vi "Test_Connection.vi"() -> ()   [LabVIEW 2024]
uses:
  <vilib>/LabVIEW Open Source Project/MQTT Control Packets/Control Packets/CONNECT/ConnectFlags -- cluster.ctl
  <vilib>/LabVIEW Open Source Project/MQTT Control Packets/Control Packets/CONNACK/Connect Return Code -- enum.ctl
  <vilib>/LabVIEW Open Source Project/MQTT Secured TCP Connection/Connection.SecuredTCP/Connection.TCP-TLS.lvclass/Connection.TCP-TLS.ctl
  dcce8393-494f-4dd8-9f2c-9d268c5ade08.vi
  <vilib>/LabVIEW Open Source Project/MQTT Secured TCP Connection/Connection.SecuredTCP/Read trusted entities.vi
  <vilib>/LabVIEW Open Source Project/MQTT Secured TCP Connection/Connection.SecuredTCP/Write trusted entities.vi
  <vilib>/LabVIEW Open Source Project/MQTT Secured TCP Connection/Connection.SecuredTCP/Connection.TCP-TLS.lvclass
  C:/Program Files (x86)/National Instruments/LabVIEW 2024/vi.lib/LabVIEW Open Source Project/Connection/Connection/Connection.lvclass
  <vilib>/LabVIEW Open Source Project/MQTT Client/Client class/Client.lvclass
  C:/Program Files (x86)/National Instruments/LabVIEW 2024/vi.lib/LabVIEW Open Source Project/MQTT Connection/MQTT_Base/Base Class/MQTT_Base.lvclass
  <vilib>/G Open Source Project for LabVIEW/MQTT Broker/Server class/Server.lvclass
  <vilib>/LabVIEW Open Source Project/MQTT Connection/MQTT_Base/Base Class/MQTT_Base.lvclass
  <vilib>/LabVIEW Open Source Project/Connection/Connection.TCP/Connection.TCP.lvclass
  <vilib>/LabVIEW Open Source Project/Connection/Connection/Connection.lvclass
  <vilib>/LabVIEW Open Source Project/MQTT Control Packets/Control Packets/CONNECT/CONNECT.lvclass
  <vilib>/LabVIEW Open Source Project/MQTT Control Packets/Control Packets/CONNACK/CONNACK.lvclass
panel:
  in  "timeout (2000 ms)":i32=2000
  in  "Keep Alive (s)":u16=60
  out "certificate added":bool
  in  "address (localhost)":string="localhost"
  in  "Server private key":path
  out "Ready for SSL":bool
  out "error out":errorcluster
  out "Return Code":T1=enum."Server Unavailable"
  in  "Connect Flags":T2={"Reserved"=FALSE, "Clean Session"=TRUE, "Will Flag"=FALSE, "Will QoS 1"=FALSE, "Will QoS 2"=FALSE, "Will Retain"=FALSE, "Password Flag"=FALSE, "User Name Flag"=FALSE}
  in  "Payload":T3
  out "NbConnections":u32
  out "error server":errorcluster
  in  "Server X.509 Certificate":path
  in  "password":string
  in  "Client Private Key":path
  in  "Client X.509 Certificate":path
  in  "Port":u16=80
  in  "Address":string="localhost"
  in  "error in (no error)":errorcluster
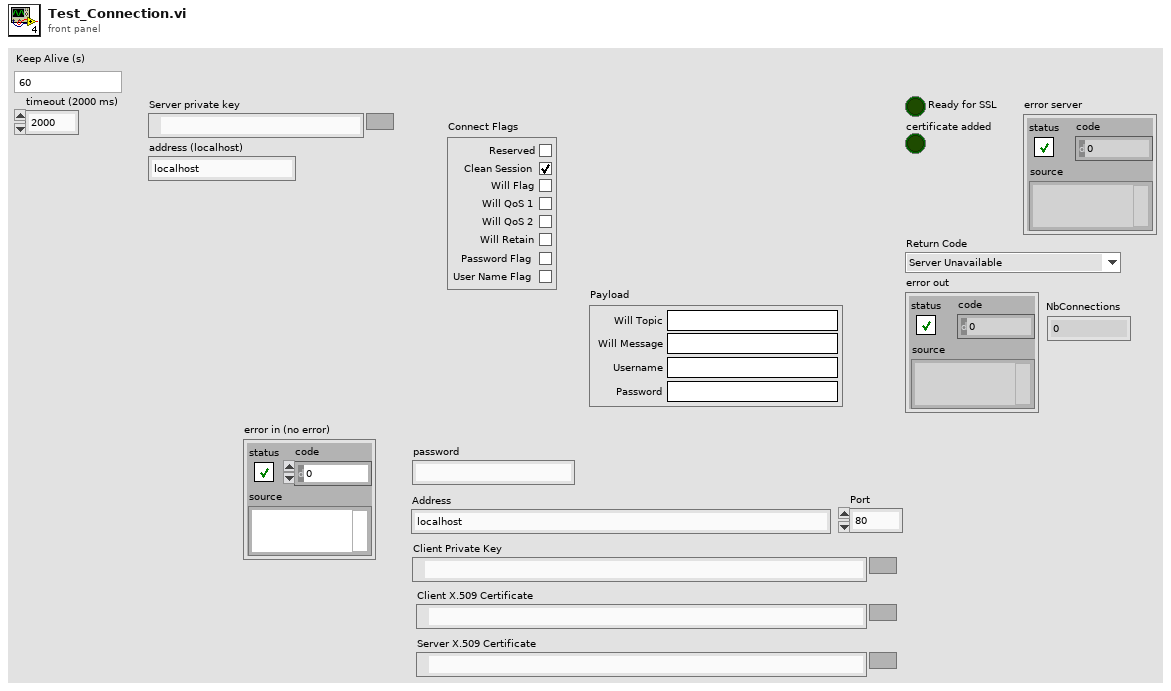
[diagram p1: front panel]
types:
  T1 = typedef "MQTT_Control_Packets.lvlib/CONNACK.lvclass/Connect Return Code -- enum.ctl" = enum16{"Connection accepted", "Unacceptable protocol version", "Identifier Rejected", "Server Unavailable", "Bad Username or Password", "Not Authorized"}
  T2 = typedef "MQTT_Control_Packets.lvlib/CONNECT.lvclass/ConnectFlags -- cluster.ctl" = cluster{"Reserved":bool, "Clean Session":bool, "Will Flag":bool, "Will QoS 1":bool, "Will QoS 2":bool, "Will Retain":bool, "Password Flag":bool, "User Name Flag":bool}
  T3 = cluster{"Will Topic":string, "Will Message":string, "Username":string, "Password":string}
  T4 = typedef "MQTT Server.lvlib/Server.lvclass/Public Events -- cluster.ctl" = cluster{"NbConnections":refnum<user-event>, "Client Event":refnum<user-event>}
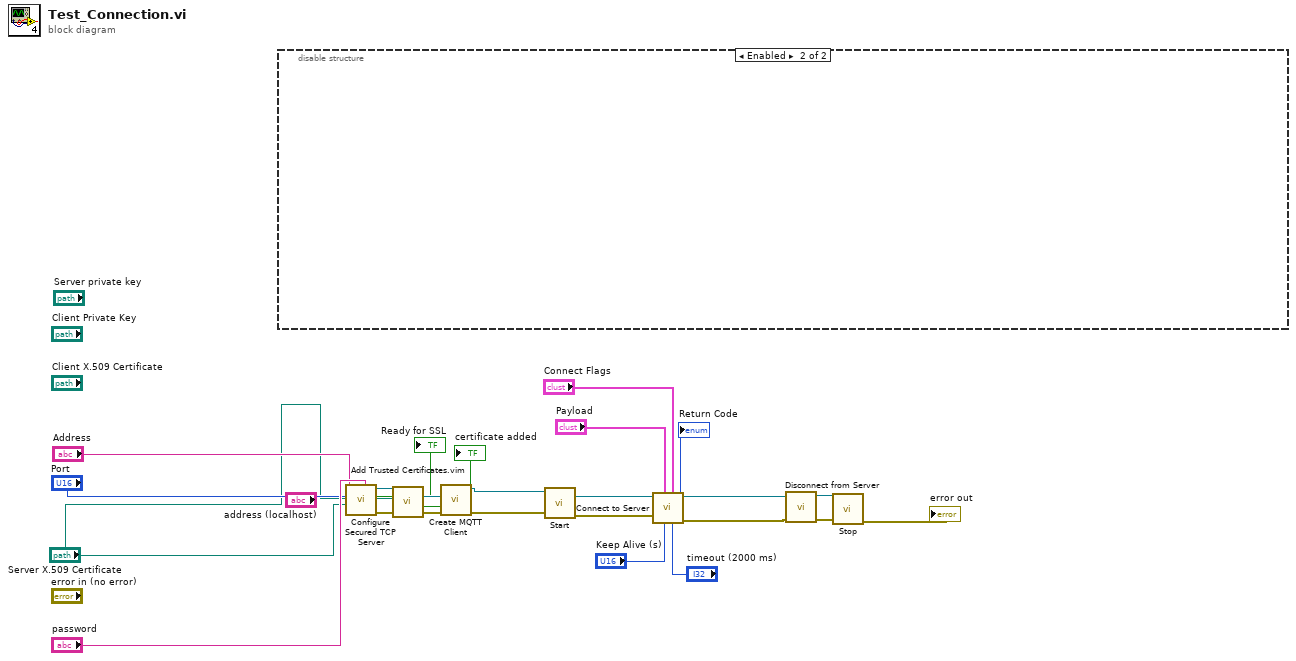
[diagram p0: block diagram]
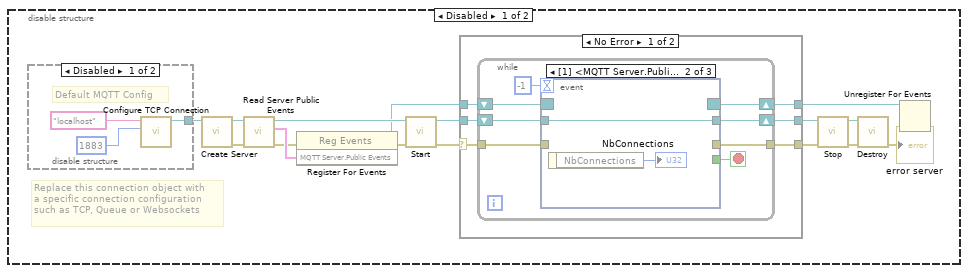
[diagram p2: hidden frame]
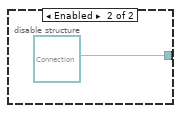
[diagram p3: hidden frame]
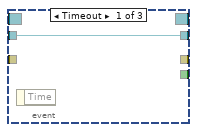
[diagram p4: hidden frame]
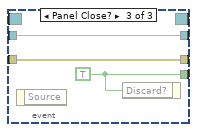
[diagram p5: hidden frame]
diagram:
  n1 = disable-structure shown="Enabled" {
    frame Disabled {
      # "Replace this connection object with\na specific connection configuration\nsuch as TCP, Queue or Websockets"
      n2 = disable-structure shown="Disabled" {
        disable-tunnel: [w41 refnum<class "Connection.lvclass"> refnum ("Connection in")] -> w40
        frame Disabled {
          # "Default MQTT Config"
          n3 = call <vilib>:"Configure TCP Connection.vi"("remote port (80)"=u16 1883, "address (localhost)"="localhost") -> ("Connection.TCP"=w41:refnum<class "Connection.TCP.lvclass">)  [unwired: 8 in, 1 out]
        }
        frame Enabled {
        }
      }
      n4 = call <vilib>:"Create Server.vi"("Connection Configuration"=w40) -> ("error out"=w26:errorcluster, "Server"=w25:refnum<class "Server.lvclass">)  [unwired: 9 in]
      n5 = call <vilib>:"Read Server Public Events.vi"("error in (no error)"=w26, "Server in"=w25) -> ("error out"=w27:errorcluster, "MQTT Server.Public Events"=w28:T4, "Server out"=w31:refnum<class "Server.lvclass">)  [unwired: 7 in]
      n6 = register-events(error in=w27, w28) -> (reference out=w29:refnum<event-registration>, error out=w33:errorcluster)  [unwired: 1 in]
      n7 = call <vilib>:"Start.vi"("error in (no error)"=w33, "MQTT_Base in"=w31) -> ("error out"=w34:errorcluster, "MQTT_Base out"=w32:refnum<class "Server.lvclass">)  [unwired: 7 in, 1 out]
      n8 = case shown="No Error" w34 {
        selector: w34 -> [w45 w65]
        tunnel: w32 -> [w50 w67]
        tunnel: [w49 w67] -> w37
        tunnel: w29 -> [w48 w66]
        tunnel: [w47 w66] -> w30
        tunnel: [w46 w65] -> w39
        frame No Error {
          n9 = while {
            shift-right: [w55] -> w49
            shift-left: w50 -> [w57]
            tunnel: [w52] -> w46
            tunnel: w45 -> [w51]
            shift-right: [w53] -> w47
            shift-left: w48 -> [w54]
            stop <- w56 stop-if-true
            n10 = event shown="[1] <MQTT Server.Public Events.NbConnections>: User Event" {
              selector: w54 -> [_ _ _]
              dyn-events: [_ _ _] -> w53
              timeout: -1 -> [_ _ _]
              tunnel: w57 -> [w59 w61 w64]
              tunnel: [_ _ w62] -> w56
              tunnel: [w59 w61 w64] -> w55
              tunnel: [_ _ w63] -> w52
              tunnel: w51 -> [_ _ w63]
              event Timeout {
                n11 = event-data() -> ()  [unwired: 1 in, 1 out]
              }
              event User Event {
                n12 = event-data() -> ("NbConnections"=→"NbConnections":u32)  [unwired: 1 in]
              }
              event Panel Close? {
                w62 = TRUE ("Discard?")
                n13 = event-data() -> ()  [unwired: 1 in, 1 out]
                n14 = event-data("Discard?"=w62) -> ()  [unwired: 1 in, 1 out]
              }
            }
          }
        }
        frame Error {
        }
      }
      n15 = call <vilib>:"Stop.vi"("error in (no error)"=w39, "MQTT_Base in"=w37) -> ("error out"=w38:errorcluster, "MQTT_Base out"=w36:refnum<class "Server.lvclass">)  [unwired: 7 in, 1 out]
      n16 = call <vilib>:"Destroy.vi"("error in (no error)"=w38, "MQTT_Base in"=w36) -> ("error out"=→"error server":errorcluster)  [unwired: 8 in, 1 out]
      n17 = Unregister For Events(event registration refnum=w30) -> ()  [unwired: 1 in, 1 out]
    }
    frame Enabled {
    }
  }
  n18 = call <vilib>:"Configure Secured TCP Server.vi"("password"="password", "Server X.509 Certificate"="Server X.509 Certificate", "remote port (443)"="Port", "address (localhost)"="Address") -> ("error out"=w18:errorcluster, "Ready for SSL"=→"Ready for SSL":bool, "Secured TCP Connection"=w16:refnum<class "Connection.TCP-TLS.lvclass">)  [unwired: 5 in]
  n19 = call "Add Trusted Certificates.vim"("error in (no error)"=w18, "Trusted Certificate"="Server X.509 Certificate", "Connection.TCP-TLS in"=w16) -> ("error out"=w19:errorcluster, "certificate added"=→"certificate added":bool, "Connection.TCP-TLS out"=w21:refnum<class "Connection.TCP-TLS.lvclass">)  [unwired: 6 in]
  n20 = call <vilib>:"Create MQTT Client.vi"("error in (no error)"=w19, "Connection Configuration"=w21) -> ("error out"=w10:errorcluster, "Client out"=w11:refnum<class "Client.lvclass">)  [unwired: 8 in]
  n21 = call <vilib>:"Start.vi"("error in (no error)"=w10, "MQTT_Base in"=w11) -> ("error out"=w9:errorcluster, "MQTT_Base out"=w8:refnum<class "Client.lvclass">)  [unwired: 7 in, 1 out]
  n22 = call <vilib>:"Connect to Server.vi"("timeout (2000 ms)"="timeout (2000 ms)", "Connect Flags"="Connect Flags", "Keep Alive (s)"="Keep Alive (s)", "Payload"="Payload", "error in (no error)"=w9, "Client in"=w8) -> ("error out"=w5:errorcluster, "Return Code"=→"Return Code":T1, "Client out"=w4:refnum<class "Client.lvclass">)  [unwired: 2 in, 1 out]
  n23 = call <vilib>:"Disconnect from Server.vi"("error in (no error)"=w5, "Client in"=w4) -> ("error out"=w2:errorcluster, "Client out"=w3:refnum<class "Client.lvclass">)  [unwired: 7 in, 1 out]
  n24 = call <vilib>:"Stop.vi"("error in (no error)"=w2, "MQTT_Base in"=w3) -> ("error out"=→"error out":errorcluster)  [unwired: 7 in, 2 out]
